vi "Get Day Number.vi"() -> (3 "Day":i32)   [LabVIEW 2021]
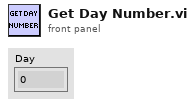
[diagram p1: front panel]
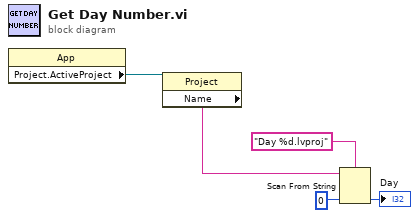
[diagram p0: block diagram]
diagram:
  n1 = property class="App"() -> ("Project.ActiveProject"=w5:refnum<vi>)  [unwired: 2 in, 2 out]
  n2 = property class="Project"(reference=w5) -> ("Name"=w4:string)  [unwired: 1 in, 2 out]
  n3 = Scan From String(format string="Day %d.lvproj", input string=w4, default 1=0) -> (output 1=→"Day":i32)  [unwired: 2 in, 3 out]
